vi "UDP - Datalogger (SubVI).vi"(6 "test?":bool, 8 "error in":errorcluster, 10 "IP":string, 11 "data in":string) -> (0 "error out":errorcluster, 3 "Channels":T1, 4 "Success":bool)   [LabVIEW 2019]
uses:
  Controls/Global - Data UDP.vi
  Controls/Global - IP Address.vi
  Controls/Global - Channel.vi
panel:
  out "Status":u8
  out "Event":u8
  out "unsigned byte array":u8[](array[numeric])
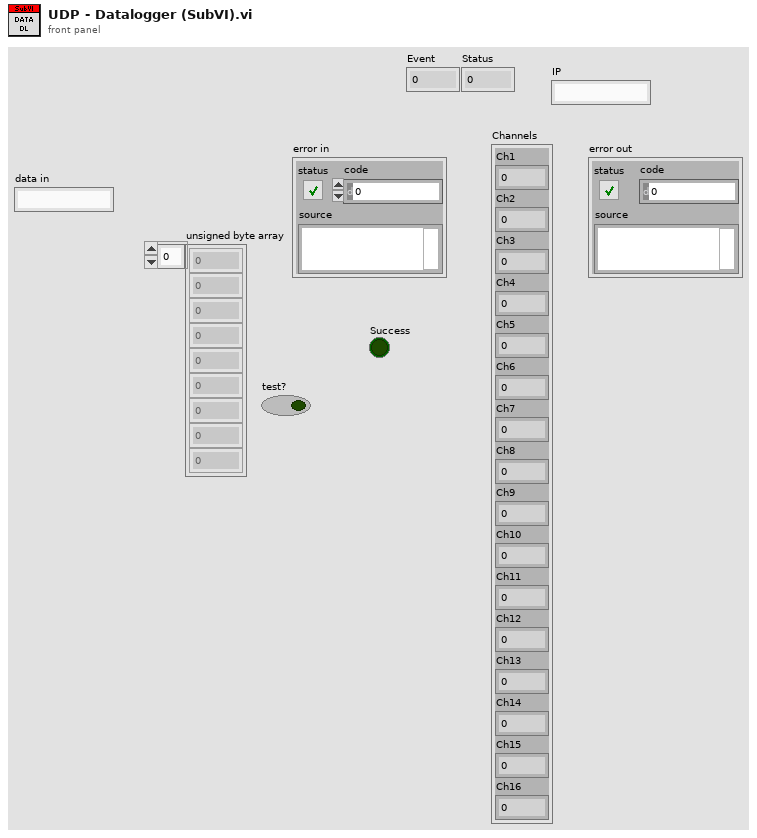
[diagram p1: front panel]
types:
  T1 = cluster{"Ch1":sgl, "Ch2":sgl, "Ch3":sgl, "Ch4":sgl, "Ch5":sgl, "Ch6":sgl, "Ch7":sgl, "Ch8":sgl, "Ch9":sgl, "Ch10":sgl, "Ch11":sgl, "Ch12":sgl, "Ch13":sgl, "Ch14":sgl, "Ch15":sgl, "Ch16":sgl}
  T2 = typedef "UDP - Event.ctl" = u16
  T3 = typedef "UDP - Status.ctl" = u16
  T4 = cluster{"Channels":cluster{"Ch1":sgl, "Ch2":sgl, "Ch3":sgl, "Ch4":sgl, "Ch5":sgl, "Ch6":sgl, "Ch7":sgl, "Ch8":sgl, "Ch9":sgl, "Ch10":sgl, "Ch11":sgl, "Ch12":sgl, "Ch13":sgl, "Ch14":sgl, "Ch15":sgl, "Ch16":sgl}, "Event":T2, "Status":T3, "IP":string}[]
  T5 = cluster{"[0]":sgl, "[1]":sgl, "[2]":sgl, "[3]":sgl, "[4]":sgl, "[5]":sgl, "[6]":sgl, "[7]":sgl, "[8]":sgl, "[9]":sgl, "[10]":sgl, "[11]":sgl, "[12]":sgl, "[13]":sgl, "[14]":sgl, "[15]":sgl}
  T6 = cluster{"Channels":cluster{"Ch1":sgl, "Ch2":sgl, "Ch3":sgl, "Ch4":sgl, "Ch5":sgl, "Ch6":sgl, "Ch7":sgl, "Ch8":sgl, "Ch9":sgl, "Ch10":sgl, "Ch11":sgl, "Ch12":sgl, "Ch13":sgl, "Ch14":sgl, "Ch15":sgl, "Ch16":sgl}, "Event":T2, "Status":T3, "IP":string}
  T7 = cluster{"Channels":cluster{"Ch1":sgl, "Ch2":sgl, "Ch3":sgl, "Ch4":sgl, "Ch5":sgl, "Ch6":sgl, "Ch7":sgl, "Ch8":sgl, "Ch9":sgl, "Ch10":sgl, "Ch11":sgl, "Ch12":sgl, "Ch13":sgl, "Ch14":sgl, "Ch15":sgl, "Ch16":sgl}, u8, u8, "IP":string}
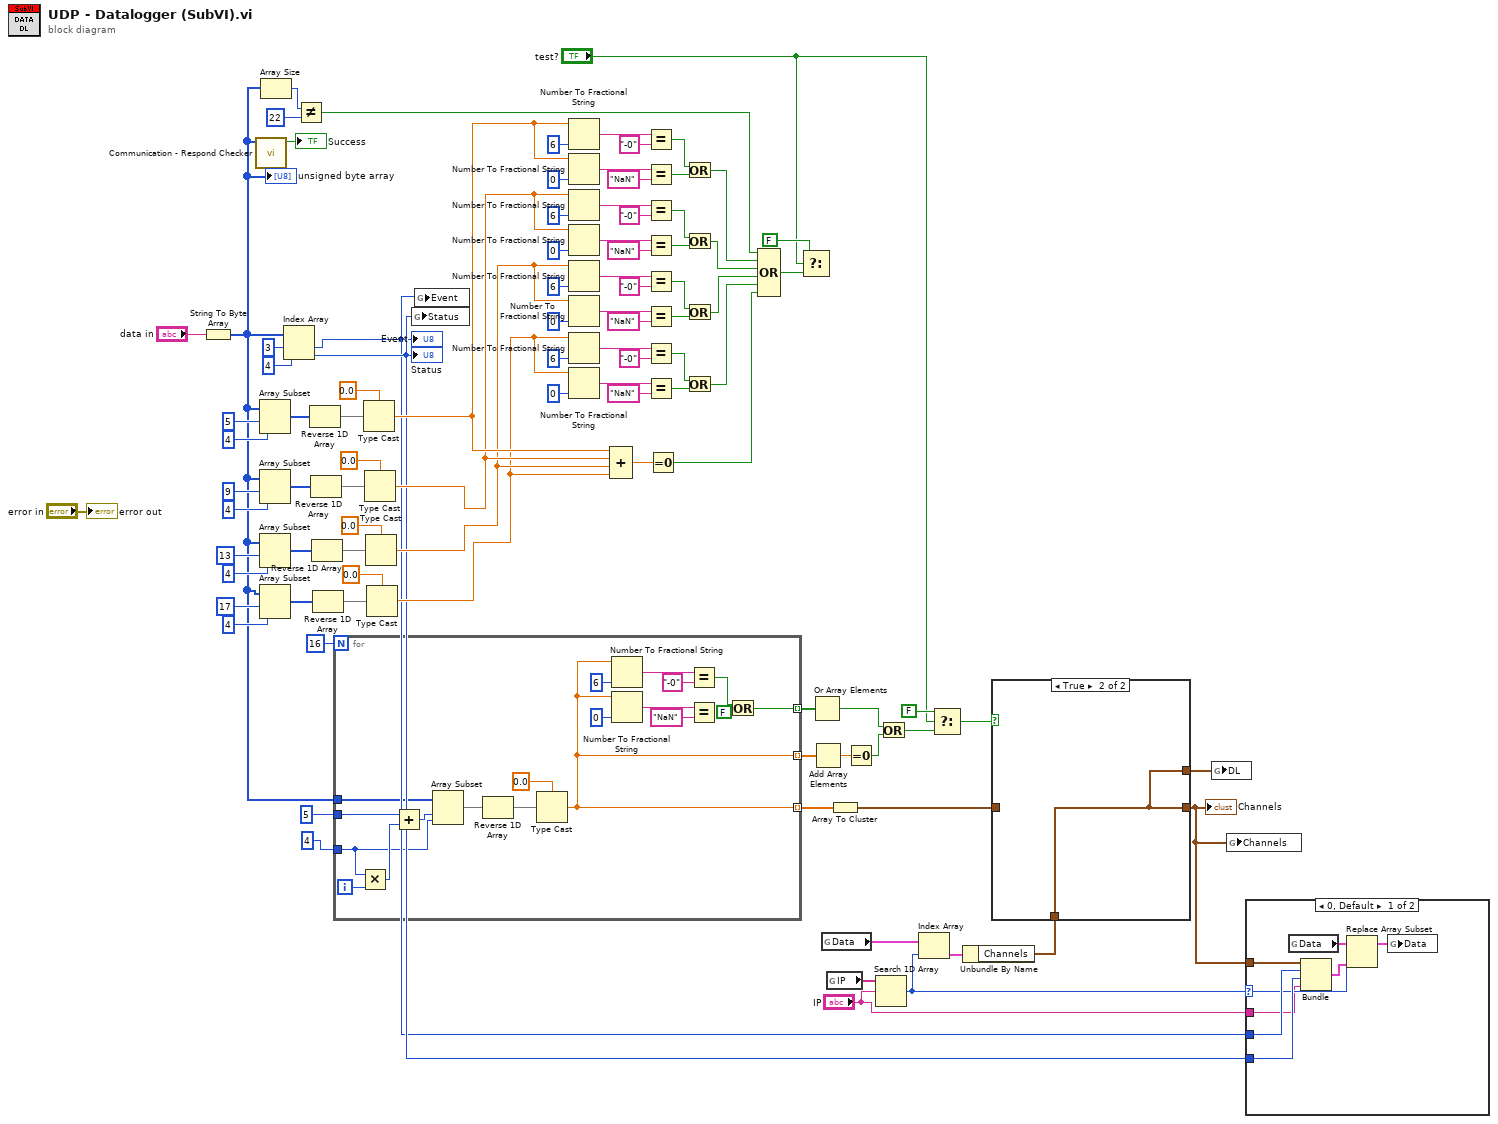
[diagram p0: block diagram]
diagram:
  n1 = String To Byte Array(string="data in") -> (unsigned byte array=w25:u8[])
  "unsigned byte array" <- w25
  n2 = call "Communication - Respond Checker.vi"("Read Data"=w25) -> ("Success"=→"Success":bool)  [unwired: 10 in]
  n3 = Array Subset(array=w25, index=5, length=4) -> (w79:u8[])
  n4 = Array Subset(array=w25, index=9, length=4) -> (w93:u8[])
  n5 = Array Subset(array=w25, index=13, length=4) -> (w94:u8[])
  n6 = Array Subset(array=w25, index=17, length=4) -> (w95:u8[])
  n7 = Array Size(array=w25) -> (size(s)=w36:i32)
  n8 = Index Array(array=w25, index #1=3 ("index"), index #2=4 ("index")) -> (element #1=w3:u8, element #2=w4:u8)
  "Event" <- w3
  "Status" <- w4
  n9 = Not Equal?(x=w36, y=22) -> (x != y?=w34:bool)
  n10 = Reverse 1D Array(array=w79) -> (reversed array=w80:u8[])
  n11 = Reverse 1D Array(array=w93) -> (reversed array=w87:u8[])
  n12 = Reverse 1D Array(array=w94) -> (reversed array=w90:u8[])
  n13 = Reverse 1D Array(array=w95) -> (reversed array=w91:u8[])
  n14 = for {
    N: 16 -> [_]
    tunnel: w25 -> [w113]
    tunnel: 5 ("index") -> [w108]
    tunnel: 4 ("length") -> [w111]
    tunnel: [w99] -> w21 mode=indexing
    tunnel: [w100] -> w19 mode=indexing
    tunnel: [w99] -> w12 mode=indexing
    i -> [w110]
    n15 = Multiply(x=w111, y=w110) -> (x*y=w112:i32)
    n16 = Add(x=w108, y=w112) -> (x+y=w109:i32)
    n17 = Array Subset(array=w113, index=w109, length=w111) -> (w115:u8[])
    n18 = Reverse 1D Array(array=w115) -> (reversed array=w114:u8[])
    n19 = Type Cast(type=sgl 0.0, x=w114) -> (*(type *) &x=w99:sgl)
    n20 = Number To Fractional String(number=w99, precision (6)=i16 6) -> (F-format string=w102:string)  [unwired: 2 in]
    n21 = Number To Fractional String(number=w99, precision (6)=i16 0) -> (F-format string=w105:string)  [unwired: 2 in]
    n22 = Equal?(x=w102, y="-0") -> (x = y?=w107:bool)
    n23 = Equal?(x=w105, y="NaN") -> ()  [unwired: 1 out]
    n24 = Or(x=w107, y=FALSE) -> (x .or. y?=w100:bool)
  }
  n25 = Type Cast(type=sgl 0.0, x=w80) -> (*(type *) &x=w33:sgl)
  n26 = Type Cast(type=sgl 0.0, x=w87) -> (*(type *) &x=w32:sgl)
  n27 = Type Cast(type=sgl 0.0, x=w90) -> (*(type *) &x=w31:sgl)
  n28 = Type Cast(type=sgl 0.0, x=w91) -> (*(type *) &x=w30:sgl)
  n29 = global write "Global - Data UDP.vi" "Status"(w4) -> ()
  n30 = global write "Global - Data UDP.vi" "Event"(w3) -> ()
  n31 = Number To Fractional String(number=w33, precision (6)=i16 6) -> (F-format string=w71:string)  [unwired: 2 in]
  n32 = Number To Fractional String(number=w33, precision (6)=i16 0) -> (F-format string=w68:string)  [unwired: 2 in]
  n33 = Number To Fractional String(number=w32, precision (6)=i16 6) -> (F-format string=w58:string)  [unwired: 2 in]
  n34 = Number To Fractional String(number=w32, precision (6)=i16 0) -> (F-format string=w61:string)  [unwired: 2 in]
  n35 = Number To Fractional String(number=w31, precision (6)=i16 6) -> (F-format string=w55:string)  [unwired: 2 in]
  n36 = Number To Fractional String(number=w31, precision (6)=i16 0) -> (F-format string=w52:string)  [unwired: 2 in]
  n37 = Number To Fractional String(number=w30, precision (6)=i16 6) -> (F-format string=w42:string)  [unwired: 2 in]
  n38 = Number To Fractional String(number=w30, precision (6)=i16 0) -> (F-format string=w45:string)  [unwired: 2 in]
  n39 = Compound Arithmetic op=ADD(w33, w32, w31, w30) -> (w29:sgl)
  n40 = Equal?(x=w71, y="-0") -> (x = y?=w66:bool)
  n41 = Equal?(x=w68, y="NaN") -> (x = y?=w65:bool)
  n42 = Equal?(x=w58, y="-0") -> (x = y?=w63:bool)
  n43 = Equal?(x=w61, y="NaN") -> (x = y?=w64:bool)
  n44 = Equal?(x=w55, y="-0") -> (x = y?=w50:bool)
  n45 = Equal?(x=w52, y="NaN") -> (x = y?=w49:bool)
  n46 = Equal?(x=w42, y="-0") -> (x = y?=w47:bool)
  n47 = Equal?(x=w45, y="NaN") -> (x = y?=w48:bool)
  n48 = Equal To 0?(x=w29) -> (x = 0?=w28:bool)
  n49 = Or(x=w66, y=w65) -> (x .or. y?=w40:bool)
  n50 = Or(x=w63, y=w64) -> (x .or. y?=w39:bool)
  n51 = Or(x=w50, y=w49) -> (x .or. y?=w38:bool)
  n52 = Or(x=w47, y=w48) -> (x .or. y?=w37:bool)
  n53 = Compound Arithmetic op=OR(w34, w40, w39, w38, w37, w28) -> (w27:bool)
  n54 = Select(t=FALSE, s="test?", f=w27) -> ()  [unwired: 1 out]
  n55 = Or Array Elements(Boolean array=w19) -> (logical OR=w18:bool)
  n56 = Add Array Elements(numeric array=w21) -> (sum=w20:sgl)
  n57 = global read "Global - Channel.vi" "Data"() -> (w8:T4)
  n58 = global read "Global - IP Address.vi" "IP"() -> (w9:string[])
  n59 = Array To Cluster(array=w12) -> (cluster=w11:T5)
  n60 = Equal To 0?(x=w20) -> (x = 0?=w17:bool)
  n61 = Search 1D Array(1D array=w9, element="IP") -> (index of element=w2:i32)  [unwired: 1 in]
  n62 = Or(x=w18, y=w17) -> (x .or. y?=w16:bool)
  n63 = Index Array(array=w8, index=w2) -> (element=w7:T6)
  n64 = Select(t=FALSE, s="test?", f=w16) -> (s? t:f=w13:bool)
  n65 = Unbundle By Name(w7) -> ("Channels"=w6:T1)
  n66 = case shown="True" w13 {
    tunnel: [w117 w118] -> w5
    tunnel: w11 -> [w117 _]
    tunnel: [w117 w118] -> w10
    tunnel: w6 -> [_ w118]
    frame False {
    }
    frame True {
    }
  }
  "Channels" <- w5
  n67 = global write "Global - Data UDP.vi" "DL"(w10) -> ()
  n68 = global write "Global - Data UDP.vi" "Channels"(w5) -> ()
  n69 = case shown="0, Default" w2 {
    selector: w2 -> [w120 _]
    tunnel: w5 -> [w123 _]
    tunnel: w4 -> [w122 _]
    tunnel: w3 -> [w121 _]
    tunnel: "IP" -> [w119 _]
    frame 0, Default {
      n70 = global read "Global - Channel.vi" "Data"() -> (w126:T4)
      n71 = Bundle("Channels"=w123, w121, w122, "IP"=w119) -> (w125:T7)  [unwired: 1 in]
      n72 = Replace Array Subset(array=w126, new element=w125, index=w120) -> (w124:T4)
      n73 = global write "Global - Channel.vi" "Data"(w124) -> ()
    }
    frame -1 {
    }
  }
  "error out" <- "error in"
